vi "Initialize Language.vi"(8 "error in (no error)":errorcluster) -> (0 "error out":errorcluster)   [LabVIEW 2019, in "GaitDAQ UI.lvlib"]
uses:
  GaitDAQ UI.lvlib
panel:
  # "Input"
  # "Output"
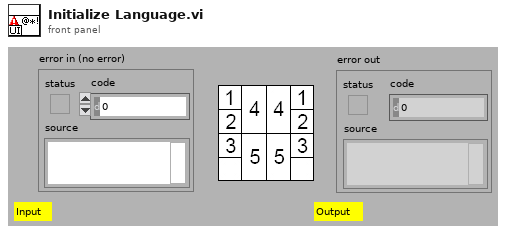
[diagram p1: front panel]
types:
  T1 = typedef "GaitDAQ UI.lvlib/UI Refnums.ctl" = cluster{"Exit Refnum":refnum<vi>}
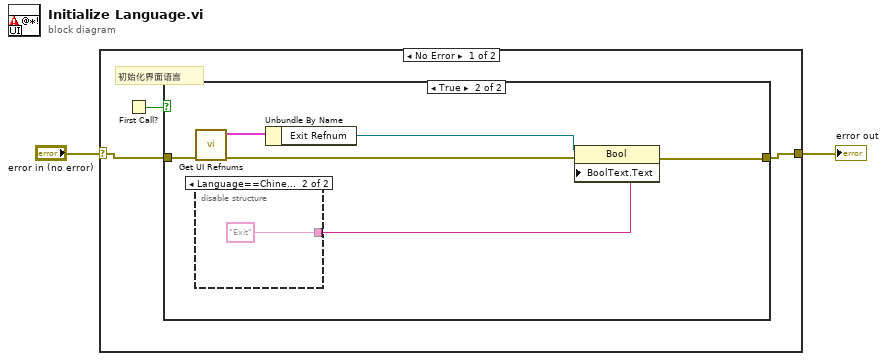
[diagram p0: block diagram]
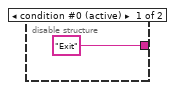
[diagram p3: hidden frame]
diagram:
  n1 = case shown="No Error" "error in (no error)" {
    selector: "error in (no error)" -> [w4 w15]
    tunnel: [w3 w15] -> w1
    frame No Error {
      # "初始化界面语言"
      n2 = First Call?() -> (First Call?: T/F=w5:bool)
      n3 = case shown="True" w5 {
        tunnel: w4 -> [w6 w12]
        tunnel: [w6 w10] -> w3
        frame False {
        }
        frame True {
          n4 = call "Get UI Refnums.vi"("error in (no error)"=w12) -> ("error out"=w7:errorcluster, "Button 0 Refnum Out"=w9:T1)  [unwired: 9 in]
          n5 = disable-structure shown="Language==Chinese" {
            disable-tunnel: ["Exit" ("Boolean Text.Text") "Exit" ("Boolean Text.Text")] -> w11
            frame condition #0 (active) {
            }
            frame condition #1 {
            }
          }
          n6 = Unbundle By Name(w9) -> ("Exit Refnum"=w8:refnum<vi>)
          n7 = property class="Bool"(reference=w8, error in=w7, "BoolText.Text"=w11) -> (error out=w10:errorcluster)  [unwired: 1 out]
        }
      }
    }
    frame Error {
    }
  }
  "error out" <- w1
